vi "countSubVIs.vi"(11 "vi path":path) -> (1 "nSubVIs":i32, 2 "Dependency Paths":path[](array[path]))   [LabVIEW 2020]
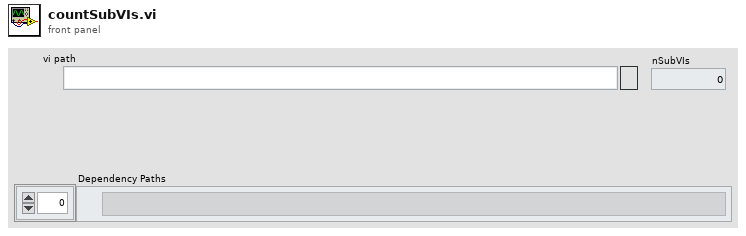
[diagram p1: front panel]
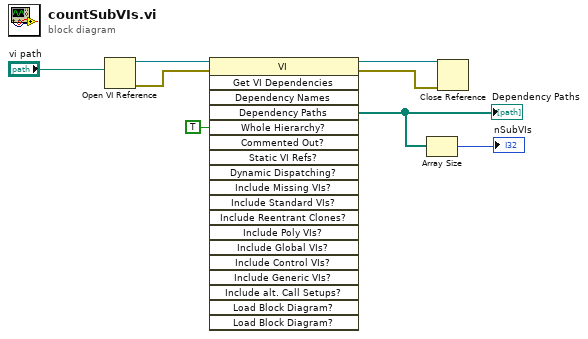
[diagram p0: block diagram]
diagram:
  n1 = Open VI Reference(vi path="vi path") -> (vi reference=w8:refnum<vi>, error out=w1:errorcluster)  [unwired: 5 in]
  n2 = invoke class="VI" method="Get VI Dependencies"(reference=w8, error in=w1, "Whole Hierarchy?"=TRUE) -> (reference out=w3:refnum<vi>, error out=w2:errorcluster, "Dependency Paths"=w6:path[])  [unwired: 16 in, 16 out]
  "Dependency Paths" <- w6
  n3 = Array Size(array=w6) -> (size(s)=→"nSubVIs":i32)
  n4 = Close Reference(reference=w3, error in (no error)=w2) -> ()  [unwired: 1 out]
